vi "xijk_get_search_table.vi"(7 "template in":u16, 8 "error in":errorcluster, 11 "Settings":T1={"search parameters"={"Paths"={"Path: Excitation filters"=path "", "Path: Dicroic filters"=path "", "Path: Emission filters"=path "", "Path reget"=path ""}, "table excitation"=[], "table dicroics"=[], "table emission"=[], "Integers"={"Select result number"=1}, "boolean selector array"=[], "table for calculation automagic"=[]}, "output cluster"={"Booleans"={"Unknown detector"=FALSE, "Dual band filters"=FALSE, "Dual emission by cubes"=FALSE, "FRET"=FALSE}, "Integers"={"Light source"=0, "Number of fluorophores"=0, "Wavelength of laser (nm) 1"=0, "Broadness of laser (nm) 1"=0.0, "Wavelength of laser (nm) 2"=0, "Broadness of laser (nm) 2"=0.0, "Template"=1}, "Doubles"={"Molar extinction 1"=1.0, "Molar extinction 2"=1.0, "Quantum efficiency 1"=1.0, "Quantum efficiency 2"=1.0}}, "output cluster 2"={"Excitation filter 1"=path "", "Dichroic filter 1"=path "", "Emission filter 1"=path "", "Excitation filter 2"=path "", "Dichroic filter 2"=path "", "Emission filter 2"=path "", "Extra em filter 1"=path "", "Extra em filter 2"=path "", "Light source file"=path "", "Fluorophore absorption 1"=path "", "Fluorophore emission 1"=path "", "Fluorophore absorption 2"=path "", "Fluorophore emission 2"=path "", "Detector"=path ""}, "cluster de sortie"={"Excitation filter_x"=[], "Excitation filter_y"=[], "Dichroic filter_x"=[], "Dichroic filter_y"=[], "Emission filter_x"=[], "Emission filter_y"=[], "Excitation filter_x 2"=[], "Excitation filter_y 2"=[], "Dichroic filter_x 2"=[], "Dichroic filter_y 2"=[], "Emission filter_x 2"=[], "Emission filter_y 2"=[], "Extra em filter_x 1"=[], "Extra em filter_y 1"=[], "Extra em filter_x 1"=[], "Extra em filter_y 2"=[], "Light source_x"=[], "Light source_y"=[], "Detector_x"=[], "Detector_y"=[], "Fluorophore absorption_x"=[], "Fluorophore absorption_y"=[], "Fluorophore emission_x"=[], "Fluorophore emission_y"=[], "Fluorophore absorption_x 2"=[], "Fluorophore absorption_y 2"=[], "Fluorophore emission_x 2"=[], "Fluorophore emission_y 2"=[], "laser_x"=[], "laser_y"=[], "laser_x 2"=[], "laser_y 2"=[], "quantum efficiency factor 1"=0.0, "quantum efficiency factor 2"=0.0}, "Xijk output cluster"={"Xijk 111"=0.0, "Xijk 112"=0.0, "Xijk 121"=0.0, "Xijk 122"=0.0, "Xijk 211"=0.0, "Xijk 212"=0.0, "Xijk 221"=0.0, "Xijk 222"=0.0, "Eijk 111"=0.0, "Eijk 112"=0.0, "Eijk 121"=0.0, "Eijk 122"=0.0, "Eijk 211"=0.0, "Eijk 212"=0.0, "Eijk 221"=0.0, "Eijk 222"=0.0}, "GUI configuration"={"axes in"={"min x-axis excitation"=300, "max x-axis excitation"=800, "min x-axis emission"=300, "max x-axis emission"=800, "precision of results"=2}, "plot colors in"={"Lanscape Portrait"=FALSE, "Plot logarithmic"=FALSE, "Ex/Em filters double"=FALSE, "Line colors"=[16734569, 56375, 16711916, 5896447, 16448250, 56375]}}, "references"={"Excitation filter 1 ref"=refnum, "Dichroic filter 1 ref"=refnum, "Emission filter 1 ref"=refnum, "Excitation filter 2 ref"=refnum, "Dichroic filter 2 ref"=refnum, "Emission filter 2 ref"=refnum, "Extra em filter 1 ref"=refnum, "Extra em filter 2 ref"=refnum, "Light source file ref"=refnum, "Fluorophore absorption 1 ref"=refnum, "Fluorophore emission 1 ref"=refnum, "Fluorophore absorption 2 ref"=refnum, "Fluorophore emission 2 ref"=refnum, "Detector ref"=refnum}} {"GUI configuration"."axes in"."precision of results" max=8 step=1}) -> (0 "error out":errorcluster, 3 "Settings out":T1={"search parameters"={"Paths"={"Path: Excitation filters"=path "", "Path: Dicroic filters"=path "", "Path: Emission filters"=path "", "Path reget"=path ""}, "table excitation"=[], "table dicroics"=[], "table emission"=[], "Integers"={"Select result number"=1}, "boolean selector array"=[], "table for calculation automagic"=[]}, "output cluster"={"Booleans"={"Unknown detector"=FALSE, "Dual band filters"=FALSE, "Dual emission by cubes"=FALSE, "FRET"=FALSE}, "Integers"={"Light source"=0, "Number of fluorophores"=0, "Wavelength of laser (nm) 1"=0, "Broadness of laser (nm) 1"=0.0, "Wavelength of laser (nm) 2"=0, "Broadness of laser (nm) 2"=0.0, "Template"=1}, "Doubles"={"Molar extinction 1"=1.0, "Molar extinction 2"=1.0, "Quantum efficiency 1"=1.0, "Quantum efficiency 2"=1.0}}, "output cluster 2"={"Excitation filter 1"=path "", "Dichroic filter 1"=path "", "Emission filter 1"=path "", "Excitation filter 2"=path "", "Dichroic filter 2"=path "", "Emission filter 2"=path "", "Extra em filter 1"=path "", "Extra em filter 2"=path "", "Light source file"=path "", "Fluorophore absorption 1"=path "", "Fluorophore emission 1"=path "", "Fluorophore absorption 2"=path "", "Fluorophore emission 2"=path "", "Detector"=path ""}, "cluster de sortie"={"Excitation filter_x"=[], "Excitation filter_y"=[], "Dichroic filter_x"=[], "Dichroic filter_y"=[], "Emission filter_x"=[], "Emission filter_y"=[], "Excitation filter_x 2"=[], "Excitation filter_y 2"=[], "Dichroic filter_x 2"=[], "Dichroic filter_y 2"=[], "Emission filter_x 2"=[], "Emission filter_y 2"=[], "Extra em filter_x 1"=[], "Extra em filter_y 1"=[], "Extra em filter_x 1"=[], "Extra em filter_y 2"=[], "Light source_x"=[], "Light source_y"=[], "Detector_x"=[], "Detector_y"=[], "Fluorophore absorption_x"=[], "Fluorophore absorption_y"=[], "Fluorophore emission_x"=[], "Fluorophore emission_y"=[], "Fluorophore absorption_x 2"=[], "Fluorophore absorption_y 2"=[], "Fluorophore emission_x 2"=[], "Fluorophore emission_y 2"=[], "laser_x"=[], "laser_y"=[], "laser_x 2"=[], "laser_y 2"=[], "quantum efficiency factor 1"=0.0, "quantum efficiency factor 2"=0.0}, "Xijk output cluster"={"Xijk 111"=0.0, "Xijk 112"=0.0, "Xijk 121"=0.0, "Xijk 122"=0.0, "Xijk 211"=0.0, "Xijk 212"=0.0, "Xijk 221"=0.0, "Xijk 222"=0.0, "Eijk 111"=0.0, "Eijk 112"=0.0, "Eijk 121"=0.0, "Eijk 122"=0.0, "Eijk 211"=0.0, "Eijk 212"=0.0, "Eijk 221"=0.0, "Eijk 222"=0.0}, "GUI configuration"={"axes in"={"min x-axis excitation"=0, "max x-axis excitation"=0, "min x-axis emission"=0, "max x-axis emission"=0, "precision of results"=0}, "plot colors in"={"Lanscape Portrait"=FALSE, "Plot logarithmic"=FALSE, "Ex/Em filters double"=FALSE, "Line colors"=[]}}, "references"={"Excitation filter 1 ref"=refnum, "Dichroic filter 1 ref"=refnum, "Emission filter 1 ref"=refnum, "Excitation filter 2 ref"=refnum, "Dichroic filter 2 ref"=refnum, "Emission filter 2 ref"=refnum, "Extra em filter 1 ref"=refnum, "Extra em filter 2 ref"=refnum, "Light source file ref"=refnum, "Fluorophore absorption 1 ref"=refnum, "Fluorophore emission 1 ref"=refnum, "Fluorophore absorption 2 ref"=refnum, "Fluorophore emission 2 ref"=refnum, "Detector ref"=refnum}} {"GUI configuration"."axes in"."precision of results" max=8 step=1})   [LabVIEW 2009]
uses:
  Type Def/settings.ctl
  Type Def/search_parameters.ctl
  Type Def/spectra_parameters.ctl
  Type Def/filepath.ctl
  Type Def/spectrum_table_control.ctl
  Type Def/xijk_cluster.ctl
  Type Def/configuration_cluster.ctl
  Type Def/axis_parameters.ctl
  Type Def/color_parameters.ctl
  Type Def/control_references_cluster.ctl
panel:
  # "Dichroic"
  # "Ex/Em filter"
  # "Fluorophore 1"
  # "Fluorophore 2"
  # "Laser /\nextra Em filter"
  # "Dichroic"
  # "Ex/Em filter"
  # "Fluorophore 1"
  # "Fluorophore 2"
  # "Laser /\nextra Em filter"
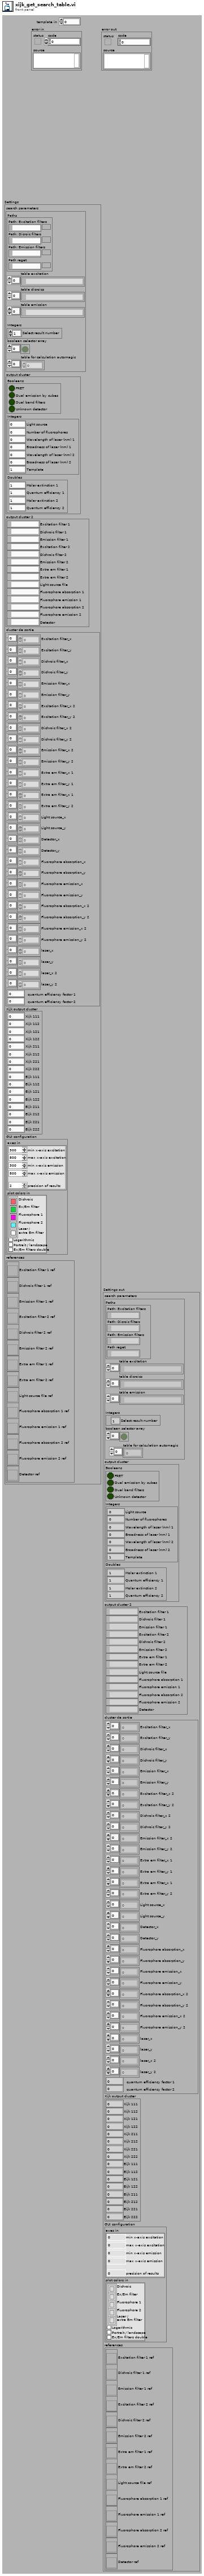
[diagram p1: front panel]
types:
  T1 = typedef "settings.ctl" = cluster{"search parameters":T2, "output cluster":T3, "output cluster 2":T4, "cluster de sortie":T5, "Xijk output cluster":T6, "GUI configuration":T7, "references":T10}
  T2 = typedef "search_parameters.ctl" = cluster{"Paths":cluster{"Path: Excitation filters":path, "Path: Dicroic filters":path, "Path: Emission filters":path, "Path reget":path}, "table excitation":path[], "table dicroics":path[], "table emission":path[], "Integers":cluster{"Select result number":u32}, "boolean selector array":bool[], "table for calculation automagic":i32[]}
  T3 = typedef "spectra_parameters.ctl" = cluster{"Booleans":cluster{"Unknown detector":bool, "Dual band filters":bool, "Dual emission by cubes":bool, "FRET":bool}, "Integers":cluster{"Light source":u16, "Number of fluorophores":u16, "Wavelength of laser (nm) 1":u16, "Broadness of laser (nm) 1":sgl, "Wavelength of laser (nm) 2":u16, "Broadness of laser (nm) 2":sgl, "Template":u16}, "Doubles":cluster{"Molar extinction 1":sgl, "Molar extinction 2":sgl, "Quantum efficiency 1":sgl, "Quantum efficiency 2":sgl}}
  T4 = typedef "filepath.ctl" = cluster{"Excitation filter 1":path, "Dichroic filter 1":path, "Emission filter 1":path, "Excitation filter 2":path, "Dichroic filter 2":path, "Emission filter 2":path, "Extra em filter 1":path, "Extra em filter 2":path, "Light source file":path, "Fluorophore absorption 1":path, "Fluorophore emission 1":path, "Fluorophore absorption 2":path, "Fluorophore emission 2":path, "Detector":path}
  T5 = typedef "spectrum_table_control.ctl" = cluster{"Excitation filter_x":i16[], "Excitation filter_y":sgl[], "Dichroic filter_x":i16[], "Dichroic filter_y":sgl[], "Emission filter_x":i16[], "Emission filter_y":sgl[], "Excitation filter_x 2":i16[], "Excitation filter_y 2":sgl[], "Dichroic filter_x 2":i16[], "Dichroic filter_y 2":sgl[], "Emission filter_x 2":i16[], "Emission filter_y 2":sgl[], "Extra em filter_x 1":i16[], "Extra em filter_y 1":sgl[], "Extra em filter_x 1":i16[], "Extra em filter_y 2":sgl[], "Light source_x":i16[], "Light source_y":sgl[], "Detector_x":i16[], "Detector_y":sgl[], "Fluorophore absorption_x":i16[], "Fluorophore absorption_y":sgl[], "Fluorophore emission_x":i16[], "Fluorophore emission_y":sgl[], "Fluorophore absorption_x 2":i16[], "Fluorophore absorption_y 2":sgl[], "Fluorophore emission_x 2":i16[], "Fluorophore emission_y 2":sgl[], "laser_x":i16[], "laser_y":sgl[], "laser_x 2":i16[], "laser_y 2":sgl[], "quantum efficiency factor 1":sgl, "quantum efficiency factor 2":sgl}
  T6 = typedef "xijk_cluster.ctl" = cluster{"Xijk 111":sgl, "Xijk 112":sgl, "Xijk 121":sgl, "Xijk 122":sgl, "Xijk 211":sgl, "Xijk 212":sgl, "Xijk 221":sgl, "Xijk 222":sgl, "Eijk 111":sgl, "Eijk 112":sgl, "Eijk 121":sgl, "Eijk 122":sgl, "Eijk 211":sgl, "Eijk 212":sgl, "Eijk 221":sgl, "Eijk 222":sgl}
  T7 = typedef "configuration_cluster.ctl" = cluster{"axes in":T8, "plot colors in":T9}
  T8 = typedef "axis_parameters.ctl" = cluster{"min x-axis excitation":u16, "max x-axis excitation":u16, "min x-axis emission":u16, "max x-axis emission":u16, "precision of results":u8}
  T9 = typedef "color_parameters.ctl" = cluster{"Lanscape Portrait":bool, "Plot logarithmic":bool, "Ex/Em filters double":bool, "Line colors":u32[]}
  T10 = typedef "control_references_cluster.ctl" = cluster{"Excitation filter 1 ref":refnum<vi>, "Dichroic filter 1 ref":refnum<vi>, "Emission filter 1 ref":refnum<vi>, "Excitation filter 2 ref":refnum<vi>, "Dichroic filter 2 ref":refnum<vi>, "Emission filter 2 ref":refnum<vi>, "Extra em filter 1 ref":refnum<vi>, "Extra em filter 2 ref":refnum<vi>, "Light source file ref":refnum<vi>, "Fluorophore absorption 1 ref":refnum<vi>, "Fluorophore emission 1 ref":refnum<vi>, "Fluorophore absorption 2 ref":refnum<vi>, "Fluorophore emission 2 ref":refnum<vi>, "Detector ref":refnum<vi>}
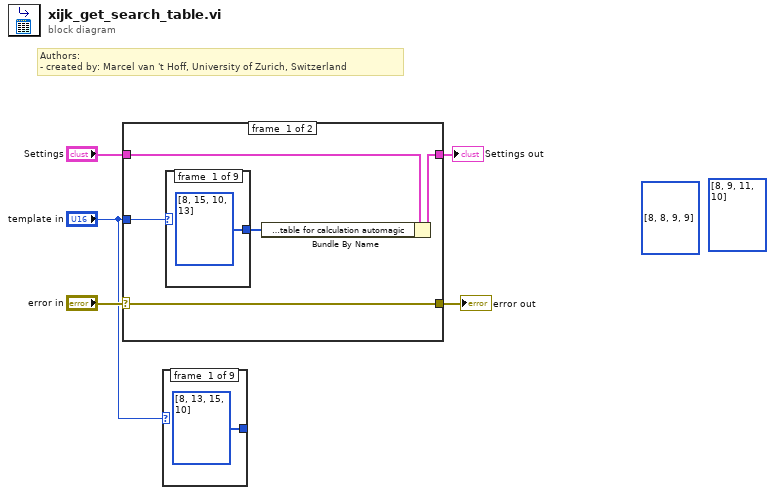
[diagram p0: block diagram]
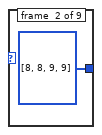
[diagram p2: hidden frame]
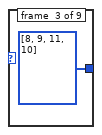
[diagram p3: hidden frame]
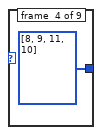
[diagram p4: hidden frame]
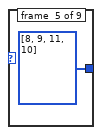
[diagram p5: hidden frame]
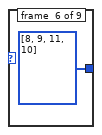
[diagram p6: hidden frame]
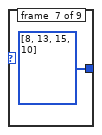
[diagram p7: hidden frame]
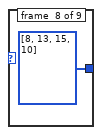
[diagram p8: hidden frame]
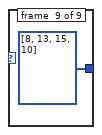
[diagram p9: hidden frame]
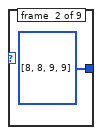
[diagram p10: hidden frame]
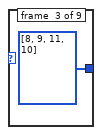
[diagram p11: hidden frame]
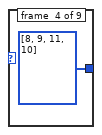
[diagram p12: hidden frame]
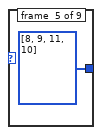
[diagram p13: hidden frame]
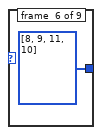
[diagram p14: hidden frame]
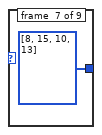
[diagram p15: hidden frame]
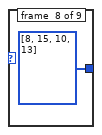
[diagram p16: hidden frame]
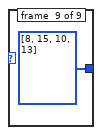
[diagram p17: hidden frame]
diagram:
  (unwired) i32[] [8, 9, 11, 10]
  (unwired) i32[] [8, 8, 9, 9]
  # "Authors: \n- created by: Marcel van 't Hoff, University of Zurich, Switzerland"
  n1 = case shown="No Error" "error in" {
    selector: "error in" -> [w9 w21]
    tunnel: "template in" -> [w10 _]
    tunnel: [w9 w21] -> w5
    tunnel: [w7 w20] -> w1
    tunnel: "Settings" -> [w8 w20]
    frame #0 {
      n2 = case shown="6" w10 {
        tunnel: [i32[] [8, 15, 10, 13] i32[] [8, 8, 9, 9] i32[] [8, 9, 11, 10] i32[] [8, 9, 11, 10] i32[] [8, 9, 11, 10] i32[] [8, 9, 11, 10] i32[] [8, 15, 10, 13] i32[] [8, 15, 10, 13] i32[] [8, 15, 10, 13]] -> w6
        frame #0 {
        }
        frame #1 {
        }
        frame #2 {
        }
        frame #3 {
        }
        frame #4 {
        }
        frame #5 {
        }
        frame #6 {
        }
        frame #7 {
        }
        frame #8 {
        }
      }
      n3 = Bundle By Name(cluster=w8, "search parameters.table for calculation automagic"=w6) -> (w7:T1)
    }
    frame #1 {
    }
  }
  "error out" <- w5
  "Settings out" <- w1
  n4 = case shown="1" "template in" {
    tunnel: [i32[] [8, 13, 15, 10] i32[] [8, 8, 9, 9] i32[] [8, 9, 11, 10] i32[] [8, 9, 11, 10] i32[] [8, 9, 11, 10] i32[] [8, 9, 11, 10] i32[] [8, 13, 15, 10] i32[] [8, 13, 15, 10] i32[] [8, 13, 15, 10]] -> _
    frame #0 {
    }
    frame #1 {
    }
    frame #2 {
    }
    frame #3 {
    }
    frame #4 {
    }
    frame #5 {
    }
    frame #6 {
    }
    frame #7 {
    }
    frame #8 {
    }
  }
